vi "TickTimeout.vi"(0 "msInicial":u32, 1 "msTimeout":u32=100000000) -> (2 "msTick":u32, 3 "msOut":u32, 4 "Timeout":bool)   [LabVIEW 2012]
panel:
  out "s? t:f":u32
  out "x > y?":bool
  # "Este VI tem comportamento diferente em função de msTimeout estar ou não conectado:\n- Se msTimeout não for conectado, msOut retorna o valor do contador de Ticks, limitado a 2^31.\n- Se msTimeout estiver conectado, o valor do contador de Ticks é subtraído de msInicial e resultado comparado com o valor de msTimeout. Se o resultado for menor que msTimeout, Timeout = 0 e \nmsOut retorna o tempo restante para atingir o timeout (msInicial + msTimeout - ContadorTicks) . Se o resultado for maior ou igual que msTimeout, Timeout = 1 e msOut retorna o tempo transcorrido depois do timeout (ContadorTicks - msInicial - msTimeout).\n- Independente de msTimeout, msTick retorna o valor do contador de Ticks.\n\nNOTA: o valor máximo permitido para msTimeout é 86400000 (número de Ticks em um dia). \n\nEste VI foi criado para tratar o overflow do contador de Ticks de 2^32 para 0."
  # "Usar este VI da seguinte forma:\nNo instante em que um período de timeout for iniciado, colocar este VI no código, sem nenhuma\nentrada conectada, e conectar a saída msTick a uma variável \"X\", que registrará o início do timeout.\nPara testar se o período de timeout foi transcorrido, colocar este VI no código, conectando a variável\n\"X\" na entrada msInicial, o valor desejado de timeout, em milisegundos, na entrada msTimeout e\ntestar a saída Timeout. Se a saída Timeout estiver setada (=1), o período de timeout foi transcorrido."
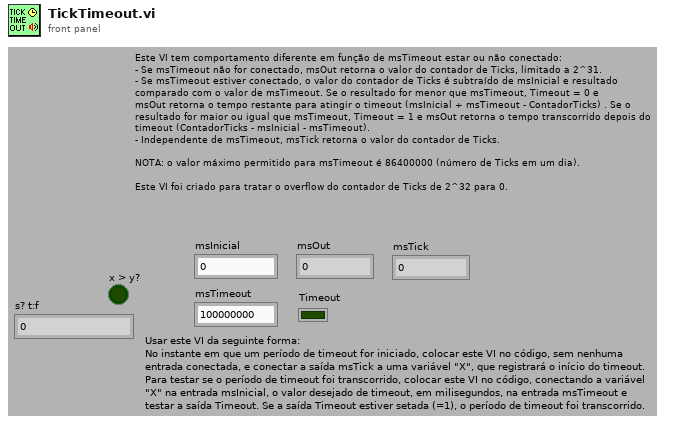
[diagram p1: front panel]
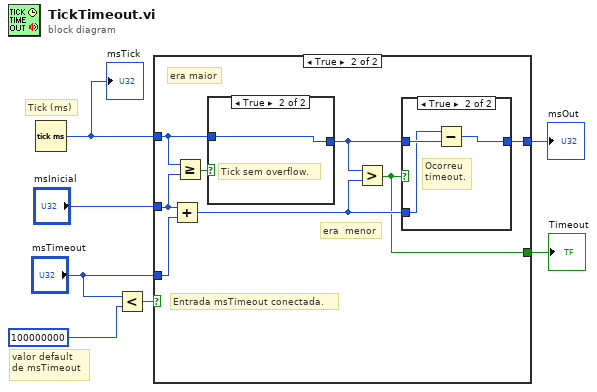
[diagram p0: block diagram]
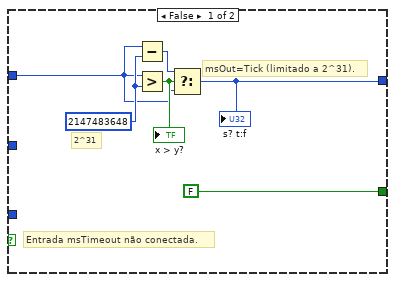
[diagram p2: hidden frame]
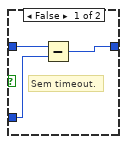
[diagram p3: hidden frame]
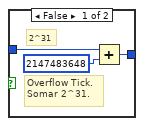
[diagram p4: hidden frame]
diagram:
  # "Tick (ms)"
  # "valor default\nde msTimeout"
  n1 = Tick Count (ms)() -> (millisecond timer value=w1:u32)
  "msTick" <- w1
  n2 = Less?(x="msTimeout", y=u32 100000000) -> (x < y?=w6:bool)
  n3 = case shown="True" w6 {
    tunnel: "msInicial" -> [_ w18]
    tunnel: "msTimeout" -> [_ w21]
    tunnel: w1 -> [w10 w19]
    tunnel: [w9 w16] -> w3
    tunnel: [FALSE w14] -> w2
    frame False {
      w12 = u32 2147483648
      # "msOut=Tick (limitado a 2^31)."
      # "Entrada msTimeout não conectada."
      # "2^31"
      n4 = Subtract(x=w10, y=w12) -> (x-y=w13:u32)
      n5 = Greater?(x=w10, y=w12) -> (0:w11:bool)
      "x > y?" <- w11
      n6 = Select(t=w13, s=w11, f=w10) -> (s? t:f=w9:u32)
      "s? t:f" <- w9
    }
    frame True {
      # "era maior"
      # "era  menor"
      # "Entrada msTimeout conectada."
      n7 = Add(x=w18, y=w21) -> (x+y=w15:u32)
      n8 = Greater Or Equal?(x=w19, y=w18) -> (x >= y?=w20:bool)
      n9 = case shown="True" w20 {
        tunnel: w19 -> [w30 w31]
        tunnel: [w28 w31] -> w17
        frame False {
          # "Overflow Tick.\nSomar 2^31."
          # "2^31"
          n10 = Add(x=w30, y=u32 2147483648) -> (x+y=w28:u32)
        }
        frame True {
          # "Tick sem overflow."
        }
      }
      n11 = Greater?(x=w17, y=w15) -> (0:w14:bool)
      n12 = case shown="True" w14 {
        tunnel: w17 -> [w24 w27]
        tunnel: [w23 w25] -> w16
        tunnel: w15 -> [w22 w26]
        frame False {
          # "Sem timeout."
          n13 = Subtract(x=w24, y=w22) -> (x-y=w23:u32)
        }
        frame True {
          # "Ocorreu\ntimeout."
          n14 = Subtract(x=w26, y=w27) -> (x-y=w25:u32)
        }
      }
    }
  }
  "msOut" <- w3
  "Timeout" <- w2
